vi "Ball Intake System.vi"(11 "Secondary Joystick Buttons":bool[](array[boolean])) -> ()   [LabVIEW 2018]
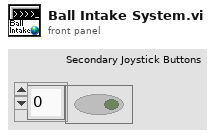
[diagram p1: front panel]
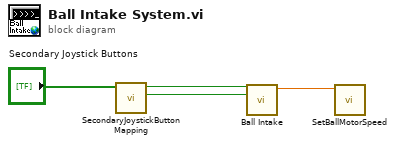
[diagram p0: block diagram]
diagram:
  n1 = call "SecondaryJoystickButtonMapping.vi"("Secondary joystick buttons"="Secondary Joystick Buttons") -> ("Outtake"=w3:bool, "Intake"=w4:bool)  [unwired: 6 in, 3 out]
  n2 = call "Ball Intake.vi"("Outtake"=w3, "Intake"=w4) -> ("IntakeSpeed"=w2:dbl)  [unwired: 9 in]
  n3 = call "SetBallMotorSpeed.vi"("IntakeSpeed"=w2) -> ()  [unwired: 11 in]
